vi "ReadJoy.vi"(5 "Teleop Local Data In":T1, 9 "error in (no error)":errorcluster) -> (6 "Teleop Local Data Out":T1, 10 "error out":errorcluster)   [LabVIEW 2019]
uses:
  Typedefs/typedef_cluster_TeleOp_Local_Data.ctl
  Typedefs/typedef_cluster_Joystick.ctl
  Typedefs/typedef_enum_refnums.ctl
  <vilib>/Rock Robotics/WPI/Utilities/WPI_GetSetVariantRefNum.vi
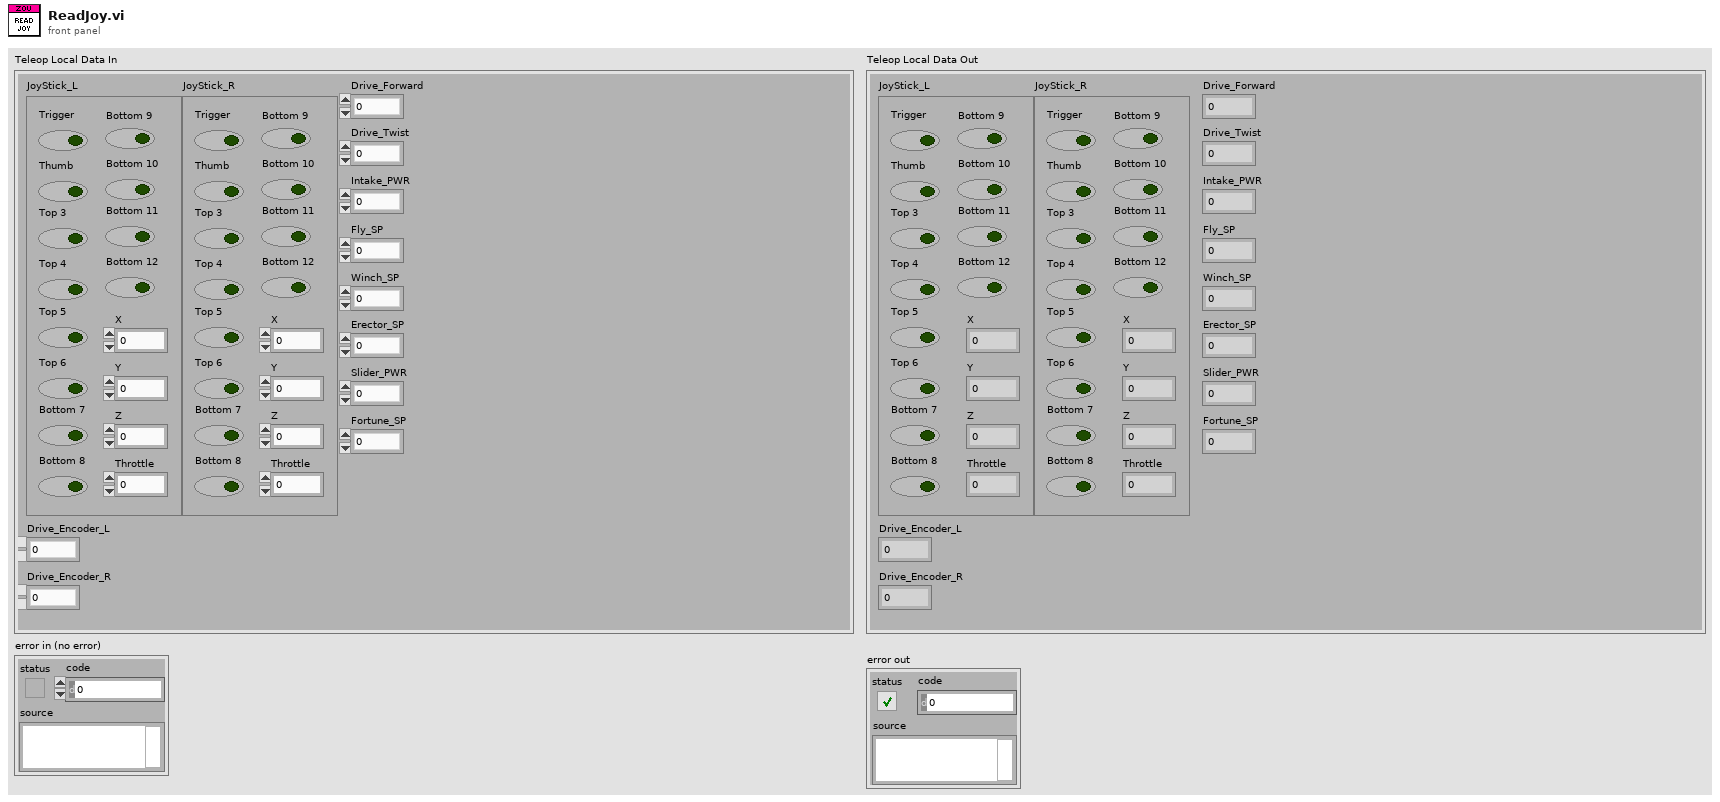
[diagram p1: front panel]
types:
  T1 = typedef "typedef_cluster_TeleOp_Local_Data.ctl" = cluster{"JoyStick_L":T2, "JoyStick_R":T2, "Drive_Forward":dbl, "Drive_Twist":dbl, "Intake_PWR":dbl, "Fly_SP":dbl, "Winch_SP":dbl, "Erector_SP":dbl, "Slider_PWR":dbl, "Fortune_SP":dbl, "Drive_Encoder_L":dbl, "Drive_Encoder_R":dbl}
  T2 = typedef "typedef_cluster_Joystick.ctl" = cluster{"X":dbl, "Y":dbl, "Z":dbl, "Throttle":dbl, "Trigger":bool, "Thumb":bool, "Top 3":bool, "Top 4":bool, "Top 5":bool, "Top 6":bool, "Bottom 7":bool, "Bottom 8":bool, "Bottom 9":bool, "Bottom 10":bool, "Bottom 11":bool, "Bottom 12":bool}
  T3 = typedef "typedef_enum_refnums.ctl" = enum16{"Joy_L", "Joy_R", "Drive_Motors", "Drive_Encoders_R", "Drive_Encoders_L", "Winch_Motor_M", "Winch_Motor_S", "Erector_Motor", "Slider_Motor", "Intake_Motor", "Fly_Motor_R", "Fly_Motor_L", "Fortune_Motor", "The_Compressor"}
  T4 = typedef "WPI_JoystickDevRef.ctl" = cluster{"Device":T5}
  T5 = typedef "WPI_JoystickDeviceEnum.ctl" = enum16{"USB 0", "USB 1", "USB 2", "USB 3", "USB 4", "USB 5"}
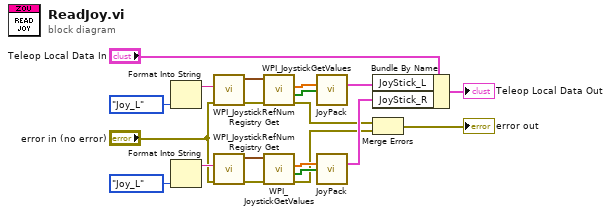
[diagram p0: block diagram]
diagram:
  n1 = Format Into String(typedef_enum_refnums."Joy_L" ("Enum")) -> (resulting string=w20:string)  [unwired: 3 in, 1 out]
  n2 = Format Into String(typedef_enum_refnums."Joy_L" ("Enum")) -> (resulting string=w13:string)  [unwired: 3 in, 1 out]
  n3 = call <vilib>:"WPI_JoystickRefNum Registry Get.vi"("error in (no error)"="error in (no error)", "refnum name"=w20) -> ("error out"=w17:errorcluster, "JoystickDevRef"=w19:T4)  [unwired: 8 out]
  n4 = call <vilib>:"WPI_JoystickRefNum Registry Get.vi"("error in (no error)"="error in (no error)", "refnum name"=w13) -> ("error out"=w16:errorcluster, "JoystickDevRef"=w14:T4)  [unwired: 8 out]
  n5 = call <vilib>:"WPI_JoystickGetValues.vi"("error in (no error)"=w17, "JoystickDevRef"=w19) -> ("error out"=w3:errorcluster, "Buttons"=w10:bool[], "Axes"=w11:dbl[])  [unwired: 5 in, 2 out]
  n6 = call <vilib>:"WPI_JoystickGetValues.vi"("error in (no error)"=w16, "JoystickDevRef"=w14) -> ("error out"=w1:errorcluster, "Buttons"=w6:bool[], "Axes"=w7:dbl[])  [unwired: 5 in, 2 out]
  n7 = call "JoyPack.vi"("Axes"=w11, "Buttons"=w10) -> ("JoyStick"=w8:T2)  [unwired: 13 in]
  n8 = call "JoyPack.vi"("Axes"=w7, "Buttons"=w6) -> ("JoyStick"=w5:T2)  [unwired: 13 in]
  n9 = Bundle By Name(cluster="Teleop Local Data In", "JoyStick_L"=w8, "JoyStick_R"=w5) -> (→"Teleop Local Data Out":T1)
  n10 = Merge Errors(w3, w1) -> (→"error out":errorcluster)
